vi "ExtractSubstring.vi"(9 "offset":i32, 11 "string byte array":u8[](array[numeric])) -> (1 "new offset":i32, 3 "sub string":string)   [LabVIEW 2017]
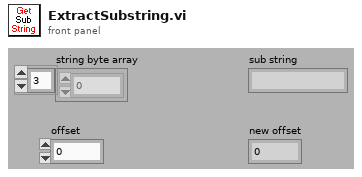
[diagram p1: front panel]
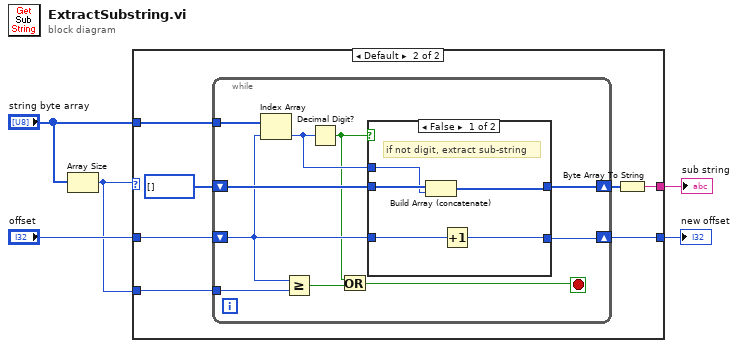
[diagram p0: block diagram]
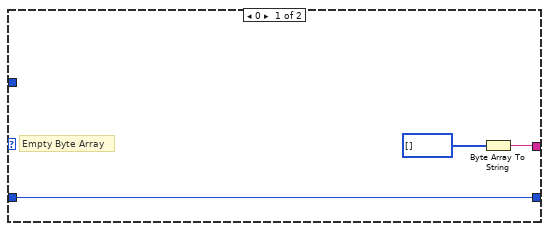
[diagram p2: hidden frame]
diagram:
  n1 = Array Size(array="string byte array") -> (size(s)=w2:i32)
  n2 = case shown="Default" w2 {
    tunnel: [w8 w13] -> w5
    tunnel: "offset" -> [w8 w14]
    tunnel: [w6 w10] -> w1
    tunnel: "string byte array" -> [_ w15]
    tunnel: w2 -> [_ w11]
    frame 0 {
      # "Empty Byte Array"
      n3 = Byte Array To String(unsigned byte array=u8[] [] ("string byte array 2")) -> (string=w6:string)
    }
    frame Default {
      n4 = while {
        tunnel: w15 -> [w25]
        shift-right: [w22] -> w13
        shift-left: w14 -> [w20]
        shift-right: [w23] -> w9
        shift-left: u8[] [] ("string byte array") -> [w24]
        tunnel: w11 -> [w19]
        stop <- w16 stop-if-true
        n5 = Index Array(array=w25, index=w20) -> (element=w21:u8)
        n6 = Greater Or Equal?(x=w20, y=w19) -> (x >= y?=w17:bool)
        n7 = Decimal Digit?(1:w21) -> (0:w18:bool)
        n8 = Or(x=w18, y=w17) -> (x .or. y?=w16:bool)
        n9 = case shown="False" w18 {
          tunnel: w24 -> [w30 w32]
          tunnel: [w28 w32] -> w23
          tunnel: [w26 w31] -> w22
          tunnel: w20 -> [w27 w31]
          tunnel: w21 -> [w29 _]
          frame False {
            # "if not digit, extract sub-string"
            n10 = Build Array (concatenate)(w30, w29) -> (w28:u8[])
            n11 = Increment(x=w27) -> (x+1=w26:i32)
          }
          frame True {
          }
        }
      }
      n12 = Byte Array To String(unsigned byte array=w9) -> (string=w10:string)
    }
  }
  "new offset" <- w5
  "sub string" <- w1
